vi "fitting_side.vi"(9 "side of clusters":cluster{"Array out":dbl[][]}[](array[cluster]), 10 "ratio":dbl, 11 "side velocity threshold":dbl) -> (1 "slope array":dbl[](array[numeric]), 2 "D of clusters":cluster{"D":ext[]}[](array[cluster]), 3 "fitting clusters":cluster{"fitting array":dbl[][]}[](array[cluster]))   [LabVIEW 2017]
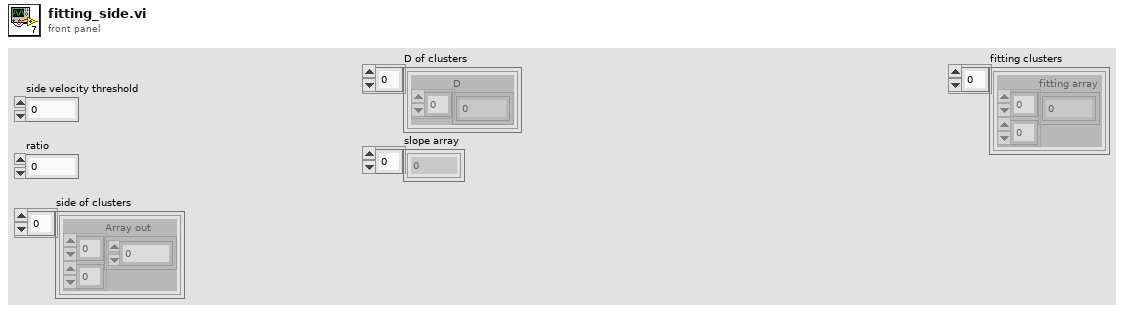
[diagram p1: front panel]
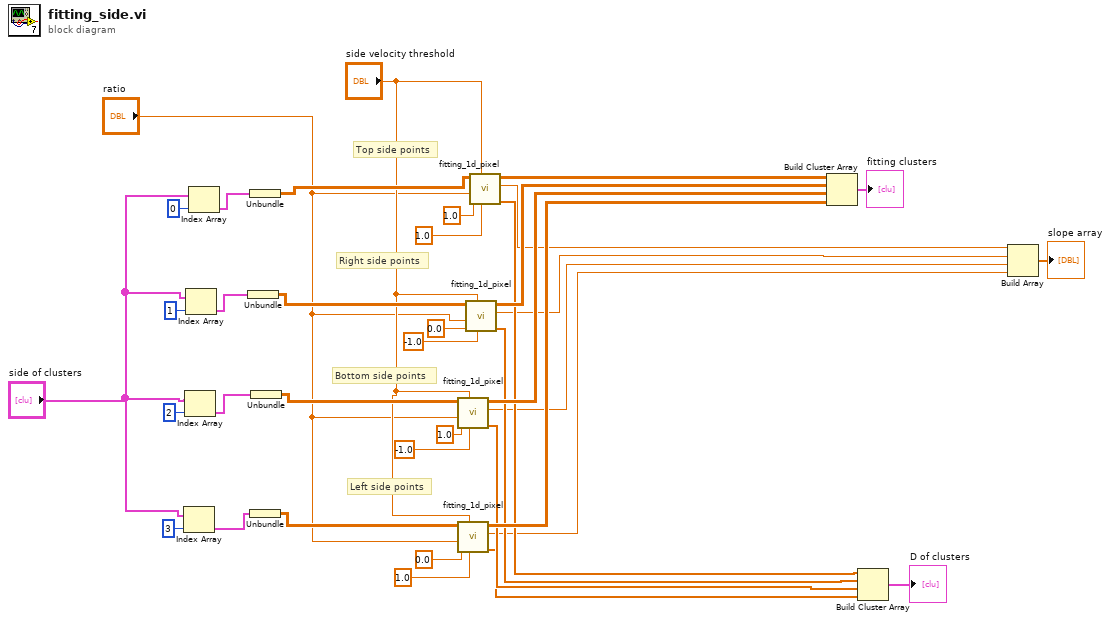
[diagram p0: block diagram]
diagram:
  # "Left side points"
  # "Bottom side points"
  # "Right side points"
  # "Top side points"
  n1 = Index Array(array="side of clusters", index=3 ("index (page)")) -> (element=w35:cluster{"Array out":dbl[][]})
  n2 = Index Array(array="side of clusters", index=2 ("index (page)")) -> (element=w34:cluster{"Array out":dbl[][]})
  n3 = Index Array(array="side of clusters", index=1 ("index (page)")) -> (element=w33:cluster{"Array out":dbl[][]})
  n4 = Index Array(array="side of clusters", index=0 ("index (page)")) -> (element=w31:cluster{"Array out":dbl[][]})
  n5 = Unbundle(w33) -> ("Array out"=w36:dbl[][])
  n6 = Unbundle(w31) -> ("Array out"=w32:dbl[][])
  n7 = Unbundle(w35) -> ("Array out"=w38:dbl[][])
  n8 = Unbundle(w34) -> ("Array out"=w37:dbl[][])
  n9 = call "fitting_1d_pixel.vi"("D sign"=-1.0, "side velocity threshold"="side velocity threshold", "fitting axis"=1.0, "ratio_pixel2mil"="ratio", "array in"=w37) -> ("D"=w8:ext[], "slope"=w3:dbl, "fitting array"=w13:dbl[][])  [unwired: 4 in]
  n10 = call "fitting_1d_pixel.vi"("D sign"=1.0, "side velocity threshold"="side velocity threshold", "fitting axis"=0.0, "ratio_pixel2mil"="ratio", "array in"=w38) -> ("D"=w7:ext[], "slope"=w1:dbl, "fitting array"=w12:dbl[][])  [unwired: 4 in]
  n11 = call "fitting_1d_pixel.vi"("D sign"=-1.0, "side velocity threshold"="side velocity threshold", "fitting axis"=0.0, "ratio_pixel2mil"="ratio", "array in"=w36) -> ("D"=w9:ext[], "slope"=w4:dbl, "fitting array"=w14:dbl[][])  [unwired: 4 in]
  n12 = call "fitting_1d_pixel.vi"("D sign"=1.0, "side velocity threshold"="side velocity threshold", "fitting axis"=1.0, "ratio_pixel2mil"="ratio", "array in"=w32) -> ("D"=w10:ext[], "slope"=w5:dbl, "fitting array"=w15:dbl[][])  [unwired: 4 in]
  n13 = Build Cluster Array(w15, w14, w13, w12) -> (→"fitting clusters":cluster{"fitting array":dbl[][]}[])
  n14 = Build Cluster Array(w10, w9, w8, w7) -> (→"D of clusters":cluster{"D":ext[]}[])
  n15 = Build Array(w5, w4, w3, w1) -> (→"slope array":dbl[])
